vi "SMO.ErrorInjection.TestLauncher.vi"() -> ()   [LabVIEW 2013, in "SMO.ErrorInjection.lvclass"]
uses:
  SMO.ErrorInjection.lvclass
  callback -- enum.ctl
  src/SMO/Typedefs/SMOState --Enum.ctl
  src/SMO/SMO.lvclass
panel:
  out "error destroy node":errorcluster
  out "error Stop node":errorcluster
  out "error Start node":errorcluster
  out "error Event Node":errorcluster
  out "error Create Node":errorcluster
  out "output cluster":errorcluster
  in  "Inject Errors":T1[](array[typedef])
  # "SMO Error Handling in Callback VIs (Test Launcher)"
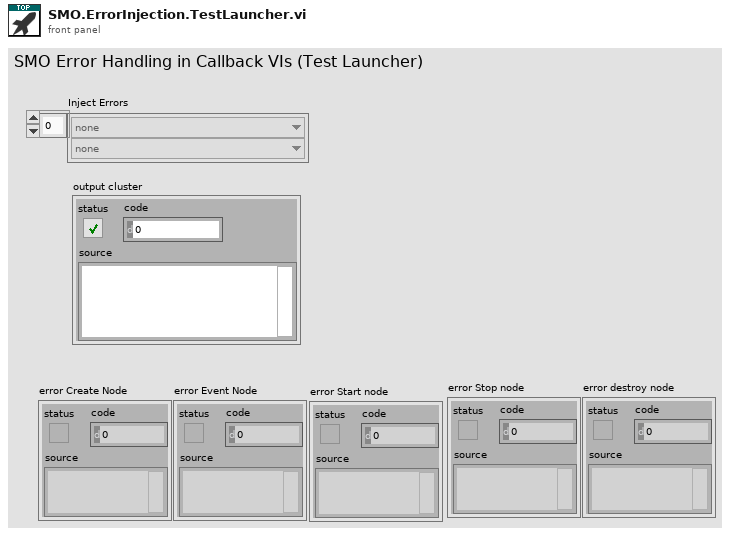
[diagram p1: front panel]
types:
  T1 = typedef "SMO.ErrorInjection.lvclass/callback -- enum.ctl" = enum16{"none", "onCreate", "onCreated", "onStart", "onStarted", "onStop", "onStopped", "onDestroy", "onDestroyed", "Handle Error", "onUnhandledDependencyError", "onDependencyMessage", "onDependencyStarted", "onDependencyStopped", "onOwnershipChanged", "enumerateStaticDependencies", "onProcessStart", "onProcessStarted", "onProcessStartedWithErrors", "onProcessStop", "onProcessStopped", "onProcessKill", "onProcessKilled"}
  T2 = typedef "SMO.lvclass/SMOState --Enum.ctl" = enum16{"unknown", "Created", "Started", "Stopped"}
  T3 = enum32{"invalid app kind", "Development System", "Run Time System", "Student Edition", "Embedded LabVIEW", "Evaluation", "Custom"}
  T4 = enum32{"Invalid", "Standard", "Closed", "Hidden", "Minimized", "Maximized"}
  T5 = cluster{"Core":cluster{"Current VI Reference":refnum<vi>, "Close Panel on Exit?":bool}, "SMO":refnum<class "SMO.ErrorInjection.lvclass">, "Your string data":string}
  T6 = cluster{"Current VI Reference":refnum<vi>, "Close Panel on Exit?":bool}
  T7 = typedef "SMO.lvclass/Public Events.ctl" = cluster{"Error":refnum<user-event>, "State":refnum<user-event>, "Reserve State":refnum<user-event>}
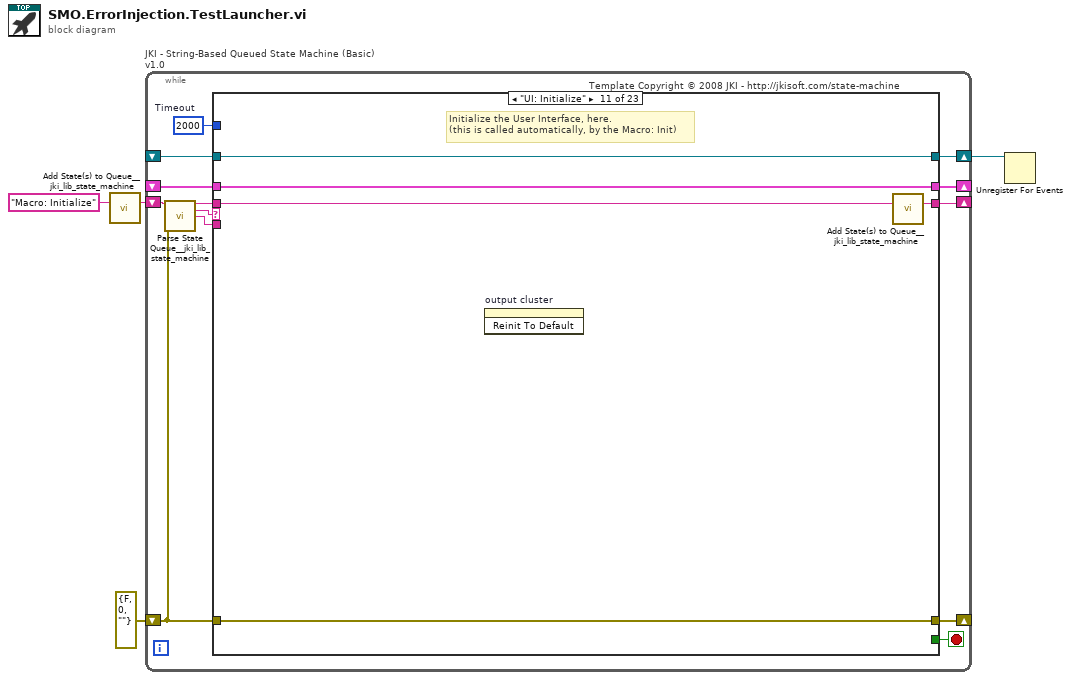
[diagram p0: block diagram]
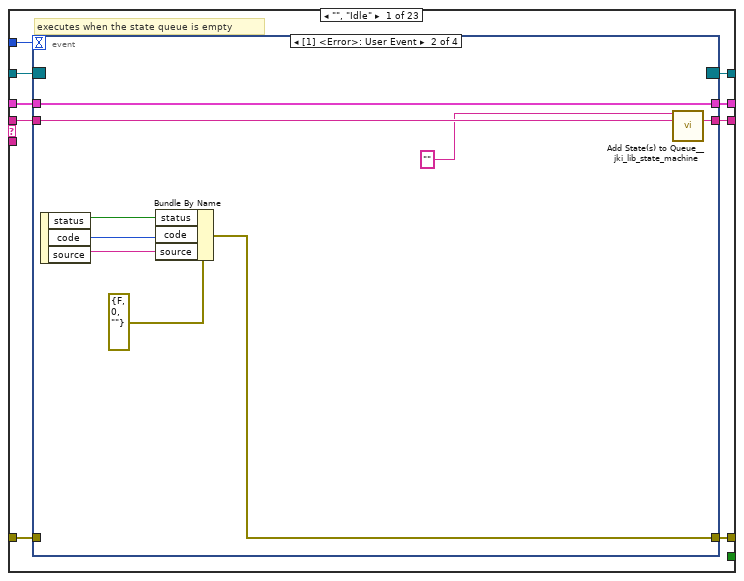
[diagram p2: hidden frame]
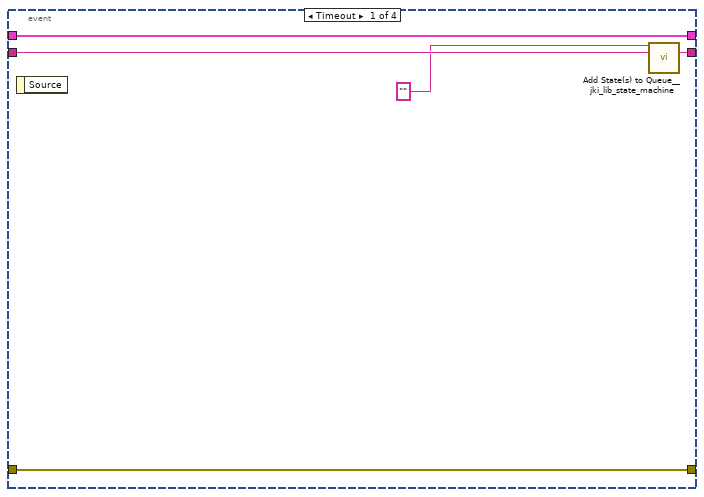
[diagram p3: hidden frame]
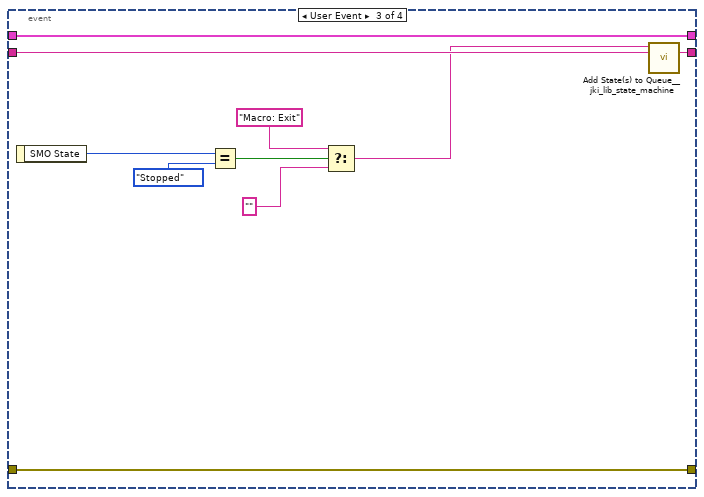
[diagram p4: hidden frame]
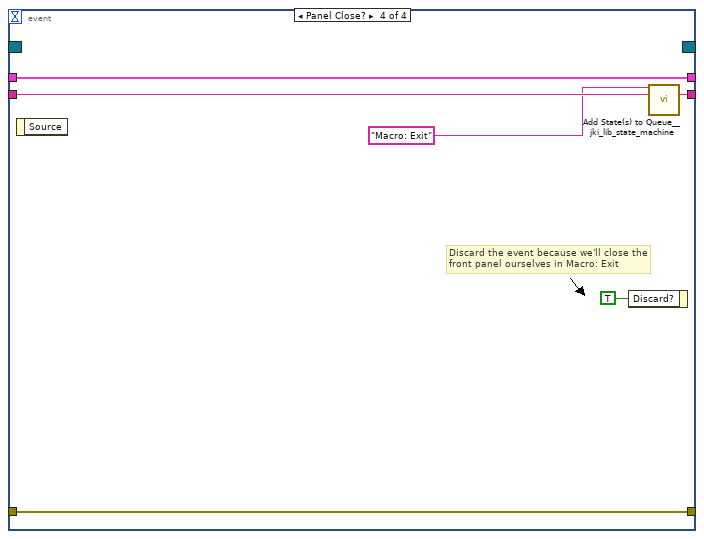
[diagram p5: hidden frame]
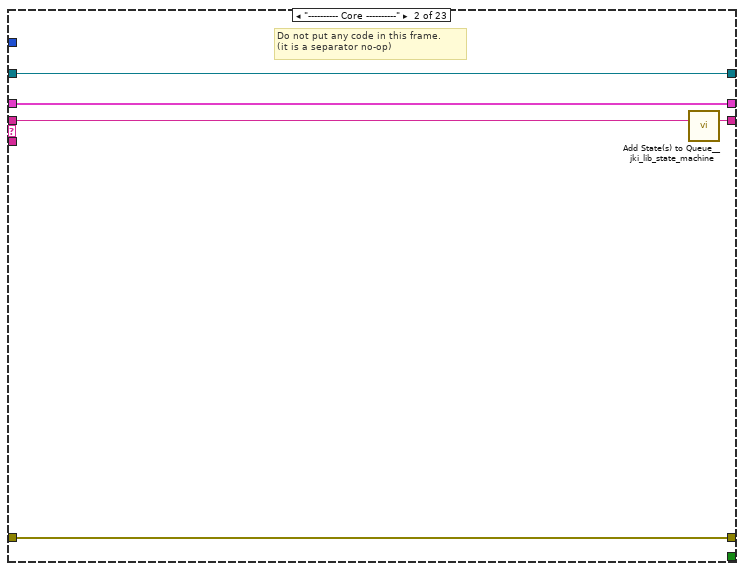
[diagram p6: hidden frame]
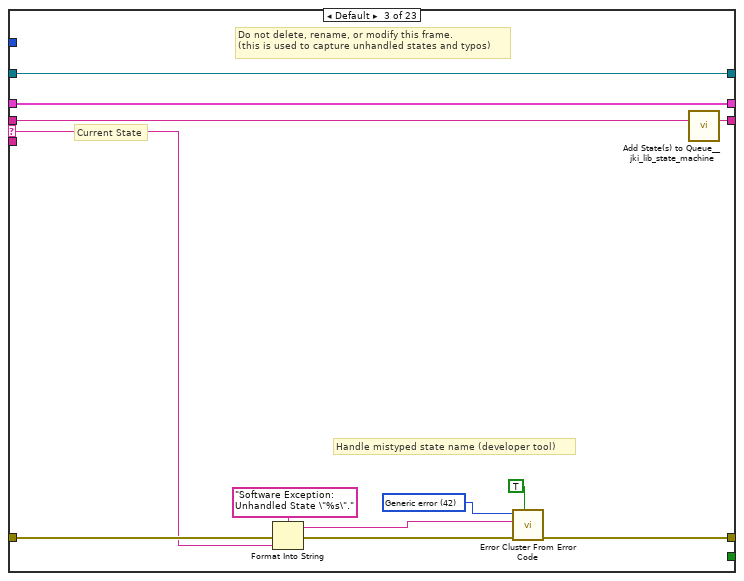
[diagram p7: hidden frame]
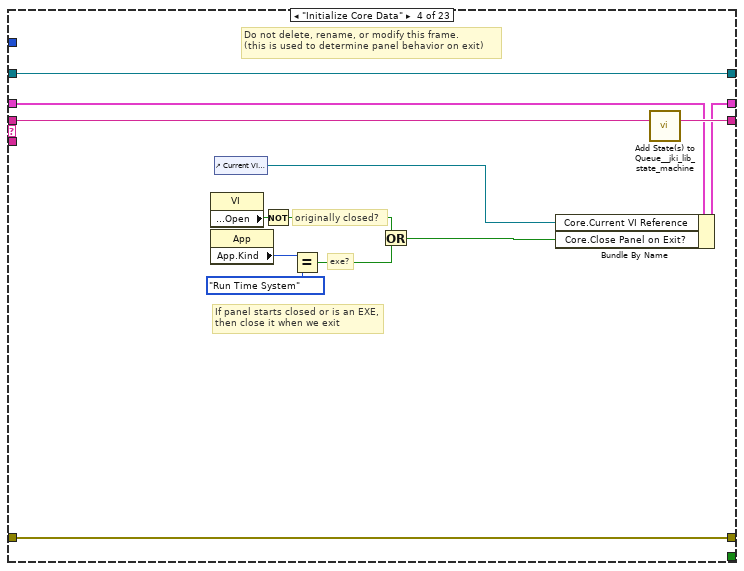
[diagram p8: hidden frame]
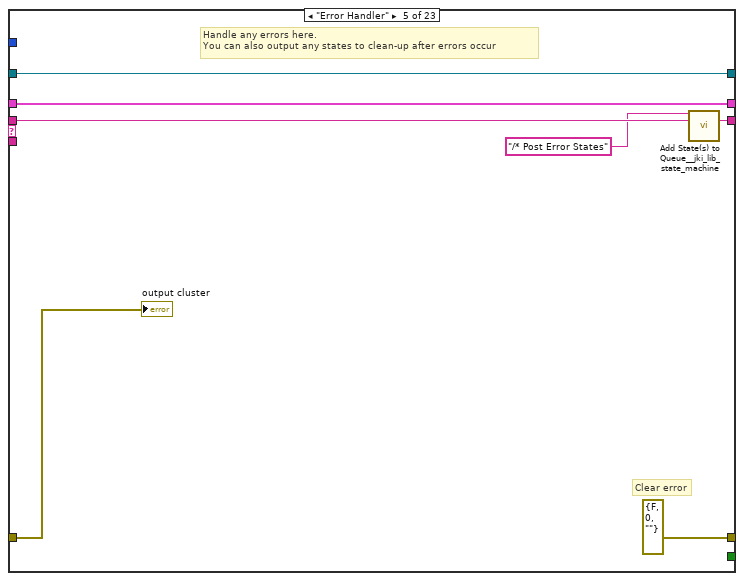
[diagram p9: hidden frame]
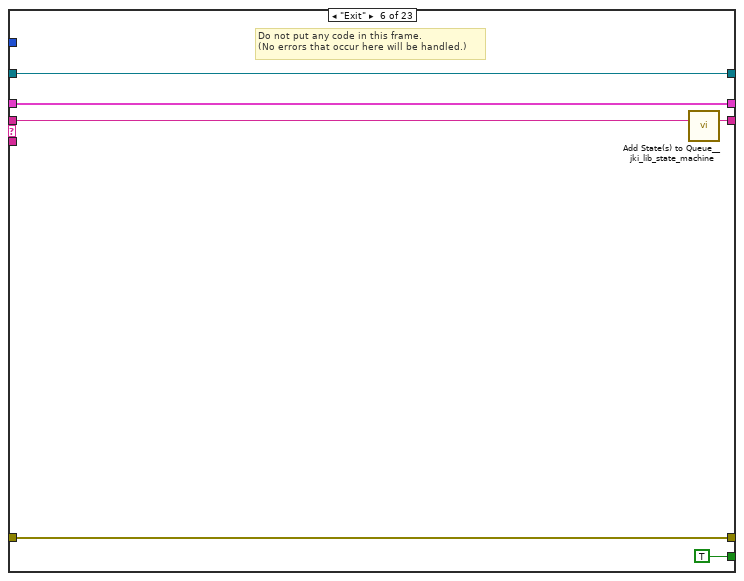
[diagram p10: hidden frame]
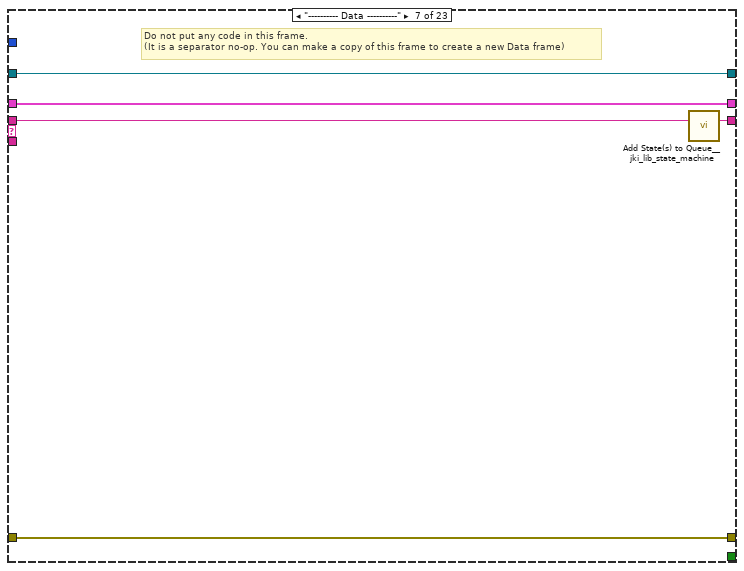
[diagram p11: hidden frame]
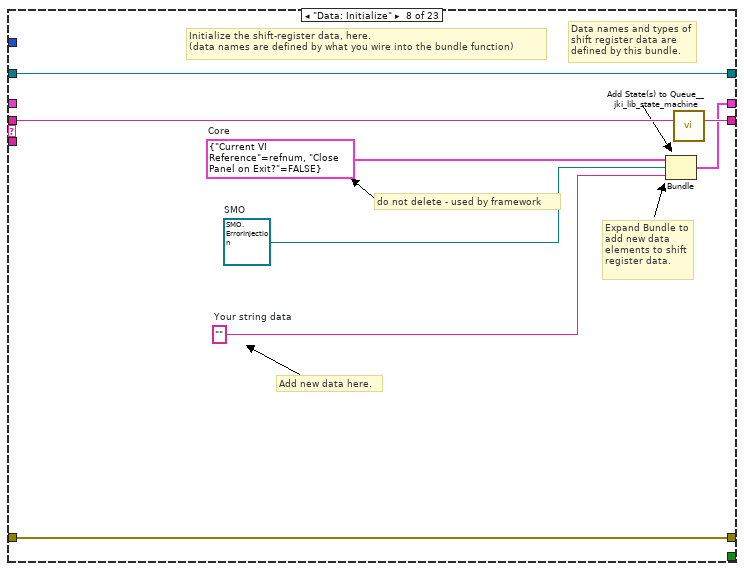
[diagram p12: hidden frame]
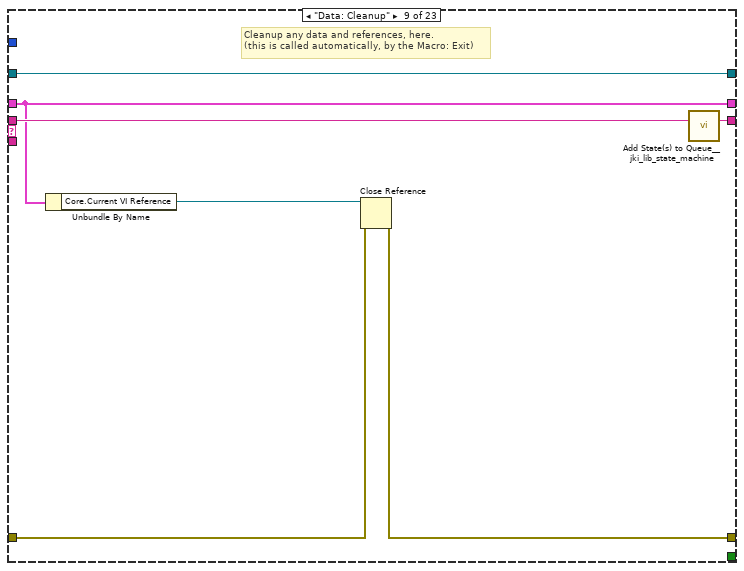
[diagram p13: hidden frame]
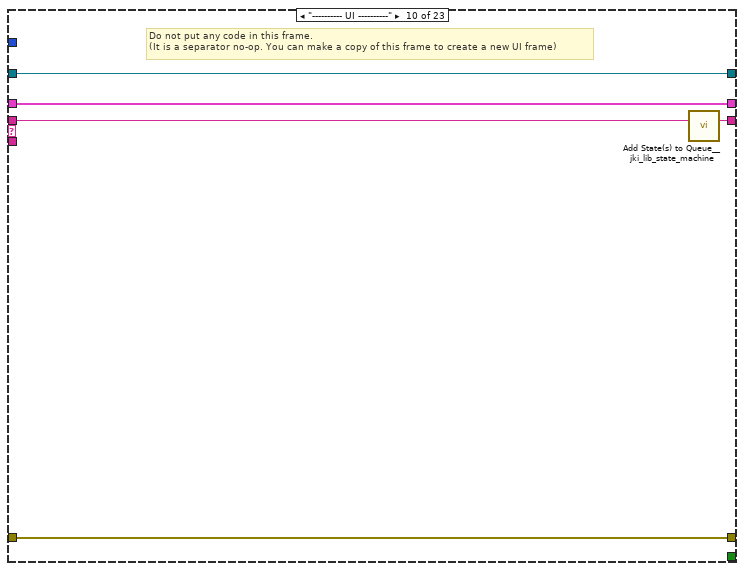
[diagram p14: hidden frame]
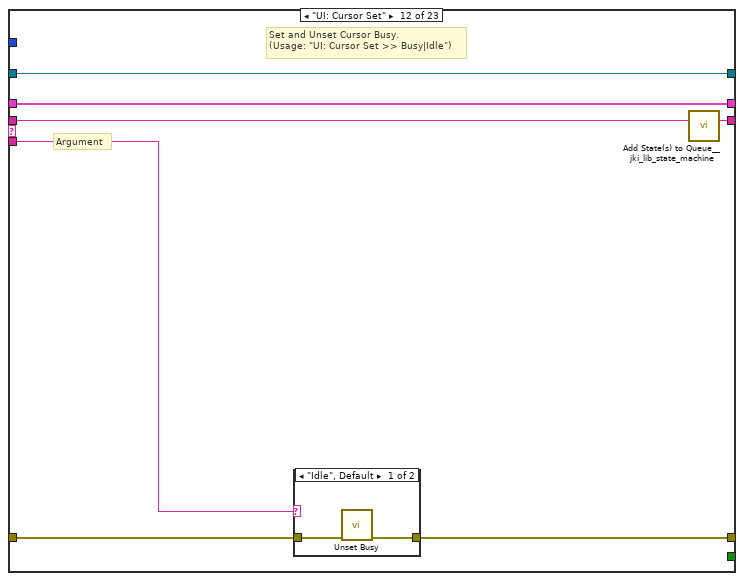
[diagram p15: hidden frame]
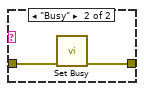
[diagram p16: hidden frame]
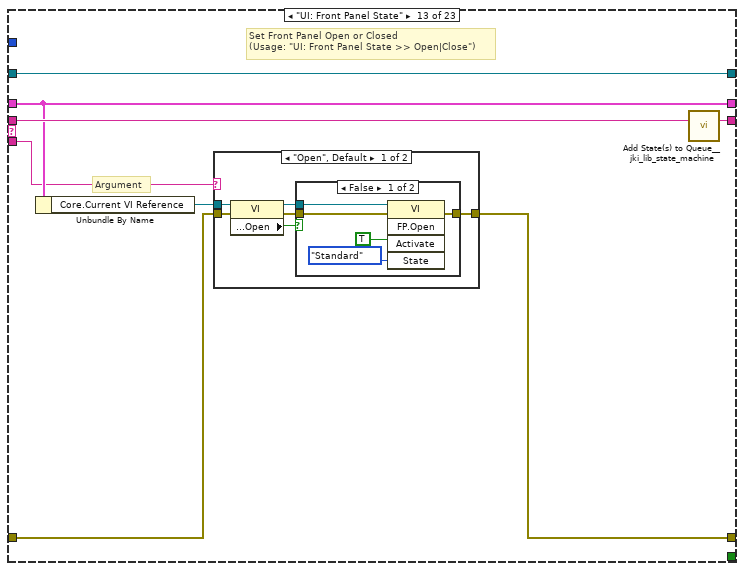
[diagram p17: hidden frame]
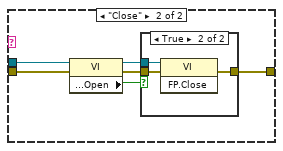
[diagram p19: hidden frame]
diagram:
  n1 = call <vilib>:"Add State(s) to Queue__jki_lib_state_machine.vi"("State(s) in (\"\")"="Macro: Initialize") -> ("States Out"=w2:string)  [unwired: 14 in]
  n2 = while "JKI - String-Based Queued State Machine (Basic) v1.0" {
    shift-right: [w10] -> _
    shift-left: _ -> [w9]
    shift-right: [w13] -> _
    shift-left: errorcluster {"status"=FALSE, "code"=0, "source"=""} ("error out") -> [w7]
    shift-right: [w12] -> _
    shift-left: w2 -> [w14]
    shift-right: [w5] -> w4
    shift-left: _ -> [w6]
    stop <- w11 stop-if-true
    w8 = 2000  # Timeout
    # "Template Copyright © 2008 JKI - http://jkisoft.com/state-machine"
    n3 = call <vilib>:"Parse State Queue__jki_lib_state_machine.vi"("State Queue"=w14, "Error In (no error)"=w7) -> ("Remaining States"=w16:string, "Current State"=w17:string, "Arguments"=w15:string)  [unwired: 11 in]
    n4 = case shown="\"UI: Initialize\"" w17 {
      selector: w17 -> [_ _ w63 _ _ _ _ _ _ _ _ _ _ _ _ _ _ _ _ _ _ _ _]
      tunnel: w16 -> [w26 w61 w67 w86 w93 w99 w104 w112 w119 w124 w129 w136 w148 w175 w181 w193 w198 w203 w208 w222 w231 w240 w249]
      tunnel: w15 -> [_ _ _ _ _ _ _ _ _ _ _ w131 w142 _ _ _ _ _ _ _ _ _ _]
      tunnel: w9 -> [w24 w58 w65 w77 w90 w97 w101 _ w114 w121 w127 w134 w144 w172 w178 w190 w195 w201 w205 w220 w227 w236 w245]
      tunnel: [w23 w59 w69 w83 errorcluster {"status"=FALSE, "code"=0, "source"=""} ("error out") w96 w102 w109 w115 w122 w126 w132 w145 w173 w179 w191 w196 w199 w206 w218 w223 w232 w242] -> w13
      tunnel: w7 -> [w22 w59 w68 w83 w87 w96 w102 w109 w116 w122 w126 w133 w146 w173 w179 w191 w196 w199 w206 w213 w224 w233 w243]
      tunnel: [w25 w60 w66 w85 w92 w98 w103 w111 w118 w123 w128 w135 w147 w174 w180 w192 w197 w202 w207 w221 w230 w239 w248] -> w12
      tunnel: [_ _ _ _ _ TRUE _ _ _ _ _ _ _ _ _ _ _ _ _ _ _ _ _] -> w11
      tunnel: [w21 w58 w65 w84 w90 w97 w101 w110 w114 w121 w127 w134 w144 w172 w178 w190 w195 w201 w205 w219 w229 w238 w247] -> w10
      tunnel: w8 -> [w20 _ _ _ _ _ _ _ _ _ _ _ _ _ _ _ _ _ _ _ _ _ _]
      tunnel: w6 -> [w19 w57 w62 w74 w88 w94 w100 w106 w113 w120 w125 w130 w141 w171 w176 w183 w194 w200 w204 _ w228 w237 w246]
      tunnel: [w18 w57 w62 w74 w88 w94 w100 w106 w113 w120 w125 w130 w141 w171 w176 w183 w194 w200 w204 w216 w228 w237 w246] -> w5
      frame "", "Idle" {
        # "executes when the state queue is empty"
        n5 = event shown="[1] <Error>: User Event" {
          selector: w19 -> [_ _ _ _]
          dyn-events: [_ _ _ _] -> w18
          timeout: w20 -> [_ _ _ _]
          tunnel: w26 -> [w31 w40 w50 w56]
          tunnel: [w30 w39 w49 w55] -> w25
          tunnel: w24 -> [w28 w38 w47 w53]
          tunnel: [w29 w32 w48 w52] -> w23
          tunnel: w22 -> [w29 _ w48 w52]
          tunnel: [w28 w38 w47 w53] -> w21
          event Timeout {
            n6 = event-data() -> ()  [unwired: 1 in, 1 out]
            n7 = call <vilib>:"Add State(s) to Queue__jki_lib_state_machine.vi"("State(s) in Front (\"\")"="", "State(s) in (\"\")"=w31) -> ("States Out"=w30:string)  [unwired: 13 in]
          }
          event User Event {
            n8 = event-data() -> ("status"=w33:bool, "code"=w34:i32, "source"=w35:string)  [unwired: 1 in]
            n9 = Bundle By Name(cluster=errorcluster {"status"=FALSE, "code"=0, "source"=""} ("error constant"), "status"=w33, "code"=w34, "source"=w35) -> (w32:errorcluster)
            n10 = call <vilib>:"Add State(s) to Queue__jki_lib_state_machine.vi"("State(s) in Front (\"\")"="", "State(s) in (\"\")"=w40) -> ("States Out"=w39:string)  [unwired: 13 in]
          }
          event User Event {
            n11 = event-data() -> ("SMO State"=w46:T2)  [unwired: 1 in]
            n12 = Equal?(x=w46, y=SMOState_--Enum."Stopped") -> (x = y?=w44:bool)
            n13 = Select(t="Macro: Exit", s=w44, f="") -> (s? t:f=w41:string)
            n14 = call <vilib>:"Add State(s) to Queue__jki_lib_state_machine.vi"("State(s) in Front (\"\")"=w41, "State(s) in (\"\")"=w50) -> ("States Out"=w49:string)  [unwired: 13 in]
          }
          event Panel Close? {
            # "Discard the event because we'll close the front panel ourselves in Macro: Exit"
            n15 = event-data() -> ()  [unwired: 1 in, 1 out]
            n16 = event-data("Discard?"=TRUE) -> ()  [unwired: 1 in, 1 out]
            n17 = call <vilib>:"Add State(s) to Queue__jki_lib_state_machine.vi"("State(s) in Front (\"\")"="Macro: Exit", "State(s) in (\"\")"=w56) -> ("States Out"=w55:string)  [unwired: 13 in]
          }
        }
      }
      frame "---------- Core ----------" {
        # "Do not put any code in this frame.\n(it is a separator no-op)"
        n18 = call <vilib>:"Add State(s) to Queue__jki_lib_state_machine.vi"("State(s) in (\"\")"=w61) -> ("States Out"=w60:string)  [unwired: 14 in]
      }
      frame Default {
        w72 = 42 items=["No error", "Argument error", "Memory is full", "Out of zone", "End of file", "File already open", "Generic file I/O error", "File not found", "File permission error", "Disk is full", "Duplicate path", "Too many files open", "System feature not enabled", "Resource file not found", "Cannot add resource", "Resource not found", "Image not found", "Image memory error", "Pen does not exist", "Config type invalid", "Config token not found", "Config parse error", "Config memory error", "Bad external code format", "Bad external code offset", "External code not present", "Null window", "Destroy window error", "Null menu", "Print aborted", "Bad print record", "Print driver error", "Windows error during printing", "Memory error during printing", "Print dialog error", "Generic print error", "Invalid device refnum", "Device not found", "Device parameter error", "Device unit error", "Cannot open device", "Device call aborted", "Generic error", "Cancelled by user", "Object ID too low", "Object ID too high", "Object not in heap", "Unknown heap", "Unknown object (invalid DefProc)", "Unknown object (DefProc not in table)", "Message out of range", "Invalid (null) method", "Unknown message", "Manager call not supported", "Bad address", "Network operation in progress", "Network operation timed out", "Connection is busy", "Network attribute not supported", "Network error", "Address in use", "System out of memory", "Connection aborted", "Connection refused", "Not connected", "Already connected", "Connection closed", "Initialization error (interapplication manager)", "Bad occurrence", "Wait on unbound occurrence handler", "Occurrence queue overflow", "Datalog type conflict", "Unused", "Unrecognized type (interapplication manager)", "Memory corrupt", "Failed to make temporary DLL", "Old CIN version", "Drag socket not found", "Failed to load drop-object", "Failed to register OLE object", "Failed to release OLE object", "Format specifier type mismatch", "Unknown format specifier", "Too few format specifiers", "Too many format specifiers", "Scan failed", "Newer CIN version", "Error converting to variant", "Runtime menu error", "Password tampered", "Variant attribute not found", "Incompatible variant data type", "Event data is not available", "Event Store is not present", "Occurrence is not found", "Event Queue is not created", "Event info is not available", "Refnum passed is NULL", "Error retrieving Class GUID", "Error retrieving CoClass GUID", "Error retrieving TypeLib GUID.", "Bad built application magic bytes.", "Specific driver is different from the specific driver associated with the Logical Name.", "There is no session opened to the class driver.", "Max Error", "MAX - Error with config objects", "MAX - Error loading configuration", "MAX - Group not supported"]
        # "Current State"
        # "Do not delete, rename, or modify this frame.\n(this is used to capture unhandled states and typos)"
        # "Handle mistyped state name (developer tool)"
        n19 = Format Into String(format string="Software Exception: Unhandled State \"%s\"." ("message"), error in=w68, w63) -> (resulting string=w71:string, error out=w70:errorcluster)  [unwired: 1 in]
        n20 = call <vilib>:"Error Cluster From Error Code.vi"("show call chain? (False)"=TRUE, "error in (no error)"=w70, "error message (\"\")"=w71, "error code (0)"=w72) -> ("error out"=w69:errorcluster)  [unwired: 5 in]
        n21 = call <vilib>:"Add State(s) to Queue__jki_lib_state_machine.vi"("State(s) in (\"\")"=w67) -> ("States Out"=w66:string)  [unwired: 14 in]
      }
      frame "Initialize Core Data" {
        # "Do not delete, rename, or modify this frame.\n(this is used to determine panel behavior on exit)"
        # "originally closed?"
        # "exe?"
        # "If panel starts closed or is an EXE, then close it when we exit"
        n22 = property class="VI"() -> ("Front Panel.Open"=w82:bool)  [unwired: 2 in, 2 out]
        n23 = property class="App"() -> ("App.Kind"=w81:T3)  [unwired: 2 in, 2 out]
        n24 = control-ref of="Current VI Reference"() -> (w75:refnum<vi>)
        n25 = Not(x=w82) -> (.not. x?=w79:bool)
        n26 = Equal?(x=w81, y=T3."Run Time System" ("Application:Kind")) -> (x = y?=w78:bool)
        n27 = Or(x=w79, y=w78) -> (x .or. y?=w76:bool)
        n28 = Bundle By Name(cluster=w77, "Core.Current VI Reference"=w75, "Core.Close Panel on Exit?"=w76) -> (w84:T5)
        n29 = call <vilib>:"Add State(s) to Queue__jki_lib_state_machine.vi"("State(s) in (\"\")"=w86) -> ("States Out"=w85:string)  [unwired: 14 in]
      }
      frame "Error Handler" {
        # "Handle any errors here.\nYou can also output any states to clean-up after errors occur"
        # "Clear error"
        n30 = call <vilib>:"Add State(s) to Queue__jki_lib_state_machine.vi"("State(s) in Front (\"\")"="/* Post Error States", "State(s) in (\"\")"=w93) -> ("States Out"=w92:string)  [unwired: 13 in]
        "output cluster" <- w87
      }
      frame "Exit" {
        # "Do not put any code in this frame.\n(No errors that occur here will be handled.)"
        n31 = call <vilib>:"Add State(s) to Queue__jki_lib_state_machine.vi"("State(s) in (\"\")"=w99) -> ("States Out"=w98:string)  [unwired: 14 in]
      }
      frame "---------- Data ----------" {
        # "Do not put any code in this frame.\n(It is a separator no-op. You can make a copy of this frame to create a new Data frame)"
        n32 = call <vilib>:"Add State(s) to Queue__jki_lib_state_machine.vi"("State(s) in (\"\")"=w104) -> ("States Out"=w103:string)  [unwired: 14 in]
      }
      frame "Data: Initialize" {
        w105 = refnum<class "SMO.ErrorInjection.lvclass"> refnum  # SMO
        w107 = T6 {"Current VI Reference"=refnum, "Close Panel on Exit?"=FALSE}  # Core
        w108 = ""  # Your string data
        # "do not delete - used by framework"
        # "Expand Bundle to add new data elements to shift register data."
        # "Add new data here."
        # "Data names and types of shift register data are defined by this bundle."
        # "Initialize the shift-register data, here.\n(data names are defined by what you wire into the bundle function)"
        n33 = Bundle("Core"=w107, "SMO"=w105, "Your string data"=w108) -> (w110:T5)  [unwired: 1 in]
        n34 = call <vilib>:"Add State(s) to Queue__jki_lib_state_machine.vi"("State(s) in (\"\")"=w112) -> ("States Out"=w111:string)  [unwired: 14 in]
      }
      frame "Data: Cleanup" {
        # "Cleanup any data and references, here.\n(this is called automatically, by the Macro: Exit)"
        n35 = Unbundle By Name(w114) -> ("Core.Current VI Reference"=w117:refnum<vi>)
        n36 = Close Reference(reference=w117, error in (no error)=w116) -> (error out=w115:errorcluster)
        n37 = call <vilib>:"Add State(s) to Queue__jki_lib_state_machine.vi"("State(s) in (\"\")"=w119) -> ("States Out"=w118:string)  [unwired: 14 in]
      }
      frame "---------- UI ----------" {
        # "Do not put any code in this frame.\n(It is a separator no-op. You can make a copy of this frame to create a new UI frame)"
        n38 = call <vilib>:"Add State(s) to Queue__jki_lib_state_machine.vi"("State(s) in (\"\")"=w124) -> ("States Out"=w123:string)  [unwired: 14 in]
      }
      frame "UI: Initialize" {
        # "Initialize the User Interface, here.\n(this is called automatically, by the Macro: Init)"
        n39 = invoke on="output cluster" class="Clust (strict)" method="Reinit To Default"() -> ()  [unwired: 3 in, 3 out]
        n40 = call <vilib>:"Add State(s) to Queue__jki_lib_state_machine.vi"("State(s) in (\"\")"=w129) -> ("States Out"=w128:string)  [unwired: 14 in]
      }
      frame "UI: Cursor Set" {
        # "Argument"
        # "Set and Unset Cursor Busy.\n(Usage: \"UI: Cursor Set >> Busy|Idle\")"
        n41 = case shown="\"Idle\", Default" w131 {
          tunnel: w133 -> [w138 w140]
          tunnel: [w137 w139] -> w132
          frame "Idle", Default {
            n42 = call <vilib>:"Unset Busy.vi"("error in (no error)"=w138) -> ("error out"=w137:errorcluster)  [unwired: 10 in]
          }
          frame "Busy" {
            n43 = call <vilib>:"Set Busy.vi"("error in (no error)"=w140) -> ("error out"=w139:errorcluster)  [unwired: 9 in, 1 out]
          }
        }
        n44 = call <vilib>:"Add State(s) to Queue__jki_lib_state_machine.vi"("State(s) in (\"\")"=w136) -> ("States Out"=w135:string)  [unwired: 14 in]
      }
      frame "UI: Front Panel State" {
        # "Argument"
        # "Set Front Panel Open or Closed\n(Usage: \"UI: Front Panel State >> Open|Close\")"
        n45 = Unbundle By Name(w144) -> ("Core.Current VI Reference"=w143:refnum<vi>)
        n46 = case shown="\"Open\", Default" w142 {
          tunnel: w146 -> [w152 w165]
          tunnel: [w154 w166] -> w145
          tunnel: w143 -> [w153 w163]
          frame "Open", Default {
            n47 = property class="VI"(reference=w153, error in=w152) -> (reference out=w150:refnum<vi>, error out=w151:errorcluster, "Front Panel.Open"=w149:bool)
            n48 = case shown="False" w149 {
              tunnel: [w157 w160] -> w154
              tunnel: w151 -> [w156 w160]
              tunnel: w150 -> [w155 _]
              frame False {
                n49 = invoke class="VI" method="FP.Open"(reference=w155, error in=w156, "Activate"=TRUE, "State"=T4."Standard") -> (error out=w157:errorcluster)  [unwired: 1 in, 4 out]
              }
              frame True {
              }
            }
          }
          frame "Close" {
            n50 = property class="VI"(reference=w163, error in=w165) -> (reference out=w162:refnum<vi>, error out=w164:errorcluster, "Front Panel.Open"=w161:bool)
            n51 = case shown="True" w161 {
              tunnel: [w167 w170] -> w166
              tunnel: w164 -> [w167 w169]
              tunnel: w162 -> [_ w168]
              frame False {
              }
              frame True {
                n52 = invoke class="VI" method="FP.Close"(reference=w168, error in=w169) -> (error out=w170:errorcluster)  [unwired: 1 in, 2 out]
              }
            }
          }
        }
        n53 = call <vilib>:"Add State(s) to Queue__jki_lib_state_machine.vi"("State(s) in (\"\")"=w148) -> ("States Out"=w147:string)  [unwired: 14 in]
      }
      frame "---------- Macro ----------" {
        # "Do not put any code in this frame.\n(It is a separator no-op. You can make a copy of this frame to create a new Macro frame)"
        n54 = call <vilib>:"Add State(s) to Queue__jki_lib_state_machine.vi"("State(s) in (\"\")"=w175) -> ("States Out"=w174:string)  [unwired: 14 in]
      }
      frame "Macro: Initialize" {
        w177 = "Data: Initialize\nInitialize Core Data\nUI: Initialize\nUI: Front Panel State >> Open\n\nTest: Create\nTest: Start\n\nMacro: Exit"  # Data: Initialize Initialize Core Data UI: Initialize UI: Front Panel State >> Open  Test: Create Test: Start  Macro: Exit
        # "Initialization Macro\n(This is called once, when the VI starts)"
        n55 = call <vilib>:"Add State(s) to Queue__jki_lib_state_machine.vi"("State(s) in Front (\"\")"=w177, "State(s) in (\"\")"=w181) -> ("States Out"=w180:string)  [unwired: 13 in]
      }
      frame "Macro: Exit" {
        # "Exit Macro\n(This is called once, when the VI exits)"
        n56 = Unbundle By Name(w190) -> ("Core.Close Panel on Exit?"=w189:bool)
        n57 = Select(t="UI: Front Panel State >> Close", s=w189, f="") -> (s? t:f=w186:string)
        n58 = call <vilib>:"Add State(s) to Queue__jki_lib_state_machine.vi"("State(s) in Front (\"\")"="Test: Stop\nTest: Destroy", "State(s) in (\"\")"=w186, "State(s) at Back (\"\")"="Data: Cleanup\nExit") -> ("States Out"=w184:string)  [unwired: 12 in]
        n59 = call <vilib>:"Add State(s) to Queue__jki_lib_state_machine.vi"("State(s) in Front (\"\")"=w184, "State(s) in (\"\")"=w193) -> ("States Out"=w192:string)  [unwired: 13 in]
      }
      frame "---------- Events ----------" {
        n60 = call <vilib>:"Add State(s) to Queue__jki_lib_state_machine.vi"("State(s) in (\"\")"=w198) -> ("States Out"=w197:string)  [unwired: 14 in]
      }
      frame "Events: Register" {
        n61 = call <vilib>:"Add State(s) to Queue__jki_lib_state_machine.vi"("State(s) in (\"\")"=w203) -> ("States Out"=w202:string)  [unwired: 14 in]
      }
      frame "---------- Test ----------" {
        n62 = call <vilib>:"Add State(s) to Queue__jki_lib_state_machine.vi"("State(s) in (\"\")"=w208) -> ("States Out"=w207:string)  [unwired: 14 in]
      }
      frame "Test: Create" {
        n63 = call "Create Error Injection Test SMO.vi"("error in (no error)"=w213, "Inject Errors"="Inject Errors") -> ("error out"=w212:errorcluster, "SMO.ErrorInjection out"=w214:refnum<class "SMO.ErrorInjection.lvclass">)  [unwired: 7 in, 1 out]
        "error Create Node" <- w212
        n64 = call "GetPublicEvents.vi"("error in (no error)"=w212, "SMO"=w214) -> ("error out"=w218:errorcluster, "Public Events"=w217:T7, "SMO out"=w211:refnum<class "SMO.ErrorInjection.lvclass">)  [unwired: 7 in]
        "error Event Node" <- w218
        n65 = Unbundle By Name(w217) -> ("State"=w215:refnum<user-event>, "Error"=w209:refnum<user-event>)
        n66 = register-events(w215, w209) -> (reference out=w216:refnum<event-registration>)  [unwired: 2 in, 1 out]
        n67 = Bundle By Name(cluster=w220, "SMO"=w211) -> (w219:T5)
        n68 = call <vilib>:"Add State(s) to Queue__jki_lib_state_machine.vi"("State(s) in (\"\")"=w222) -> ("States Out"=w221:string)  [unwired: 14 in]
      }
      frame "Test: Start" {
        n69 = Unbundle By Name(w227) -> ("SMO"=w226:refnum<class "SMO.ErrorInjection.lvclass">)
        n70 = call "Start.vi"("error in (no error)"=w224, "SMO"=w226) -> ("error out"=w223:errorcluster, "SMO out"=w225:refnum<class "SMO.ErrorInjection.lvclass">)  [unwired: 8 in]
        "error Start node" <- w223
        n71 = Bundle By Name(cluster=w227, "SMO"=w225) -> (w229:T5)
        n72 = call <vilib>:"Add State(s) to Queue__jki_lib_state_machine.vi"("State(s) in (\"\")"=w231) -> ("States Out"=w230:string)  [unwired: 14 in]
      }
      frame "Test: Stop" {
        n73 = Unbundle By Name(w236) -> ("SMO"=w235:refnum<class "SMO.ErrorInjection.lvclass">)
        n74 = call "Stop.vi"("error in (no error)"=w233, "SMO"=w235) -> ("error out"=w232:errorcluster, "SMO out"=w234:refnum<class "SMO.ErrorInjection.lvclass">)  [unwired: 8 in]
        "error Stop node" <- w232
        n75 = Bundle By Name(cluster=w236, "SMO"=w234) -> (w238:T5)
        n76 = call <vilib>:"Add State(s) to Queue__jki_lib_state_machine.vi"("State(s) in (\"\")"=w240) -> ("States Out"=w239:string)  [unwired: 14 in]
      }
      frame "Test: Destroy" {
        n77 = Unbundle By Name(w245) -> ("SMO"=w244:refnum<class "SMO.ErrorInjection.lvclass">)
        n78 = call "Destroy.vi"("error in (no error)"=w243, "SMO"=w244) -> ("error out"=w242:errorcluster)  [unwired: 9 in]
        "error destroy node" <- w242
        n79 = Bundle By Name(cluster=w245, "SMO"=refnum<class "SMO.ErrorInjection.lvclass"> refnum ("SMO.ErrorInjection.lvclass")) -> (w247:T5)
        n80 = call <vilib>:"Add State(s) to Queue__jki_lib_state_machine.vi"("State(s) in (\"\")"=w249) -> ("States Out"=w248:string)  [unwired: 14 in]
      }
    }
  }
  n81 = Unregister For Events(event registration refnum=w4) -> ()  [unwired: 1 in, 1 out]
